vi "AccelometerTest.vi"() -> ()   [LabVIEW 2014]
uses:
  <vilib>/express/express analysis/Spectral/Block/exnSpectralBlock spectral measurements RMS poly.vi
  <vilib>/express/express analysis/Spectral/Block/exnSpectralBlock spectral measurements RMS DDT.vi
  <vilib>/express/express analysis/Spectral/XNode/ExpressSpectralMeasurementsBlockNode.xnode
panel:
  out "Waveform Graph":dynamicdata(graph)
  in  "Lower Cut-Off":dbl=100.0
  out "Filtered Signal":dynamicdata(graph)
  out "data":dynamicdata(graph)
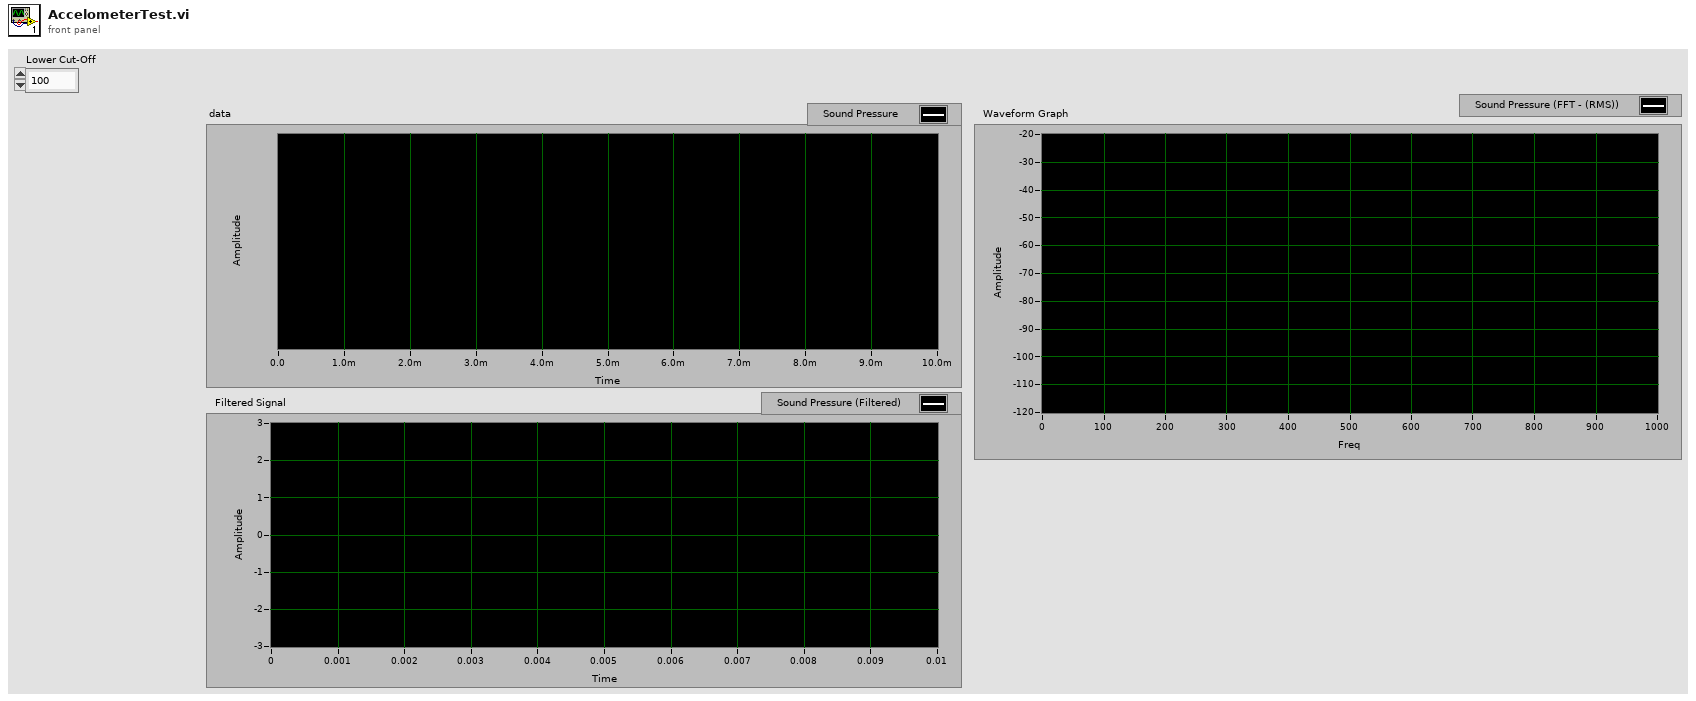
[diagram p1: front panel]
types:
  T1 = cluster{"averaging mode":u16, "weighting mode":u16, "number of averages":u32}
  T2 = cluster{"dB On (F)":bool, "unwrap phase (F)":bool, "convert to degree (F)":bool}
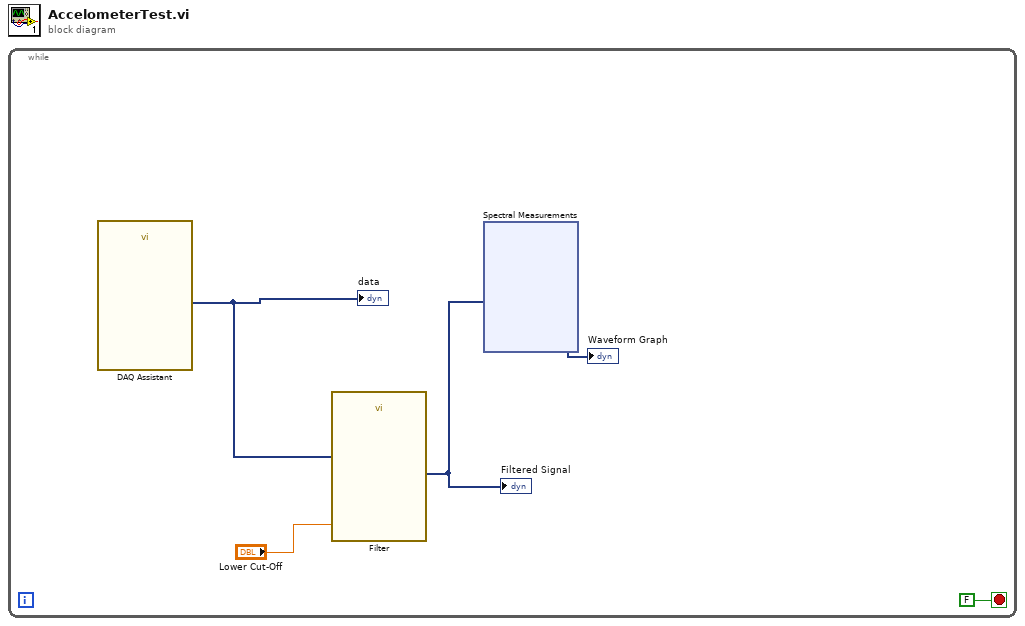
[diagram p0: block diagram]
diagram:
  n1 = while {
    stop <- FALSE ("Boolean") stop-if-true
    n2 = call "DAQ Assistant"() -> ("data"=w4:dynamicdata)  [unwired: 16 in, 3 out]
    "data" <- w4
    n3 = call "Filter"("Lower Cut-Off"="Lower Cut-Off", "Signal"=w4) -> ("Filtered Signal"=w2:dynamicdata)  [unwired: 8 in, 1 out]
    "Filtered Signal" <- w2
    n4 = xnode "Spectral Measurements"("Signals"=w2) -> ("FFT - (RMS)"=→"Waveform Graph":dynamicdata)  [unwired: 1 in, 2 out]
  }
